vi "LDA CreateEmpty.vi"(8 "error in":errorcluster, 11 "numComponents":i32) -> (0 "error out":errorcluster, 3 "LDA":refnum<class "LDA.lvclass">)   [LabVIEW 2020, in "OpenLvVision_OpenCv.lvlib" / "LDA.lvclass"]
doc: "constructor Initializes a LDA with num_components (default 0)."
uses:
  LDA.lvclass
  C:/Users/lukas/Downloads/OpenLvVision_OpenCv/SourceCode/LabView/OpenLvVision_OpenCv/_LvHelpers/EdvrObject/EdvrObject.lvclass
  _LvHelpers/EdvrObject/TypeDef/Edvr.ctl
  _LvHelpers/EdvrObject/EdvrObject.lvclass/EdvrObject.ctl
  _LvHelpers/EdvrObject/EdvrObject.lvclass
  OpenLvVision_OpenCv.lvlib
  Dlls/OlvOpenCvWrapper.dll
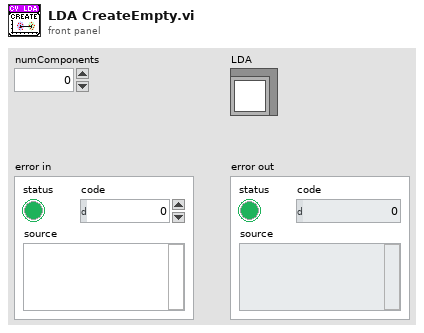
[diagram p1: front panel]
types:
  T1 = typedef "OpenLvVision_OpenCv.lvlib/EdvrObject.lvclass/Edvr.ctl" = refnum<data-value>
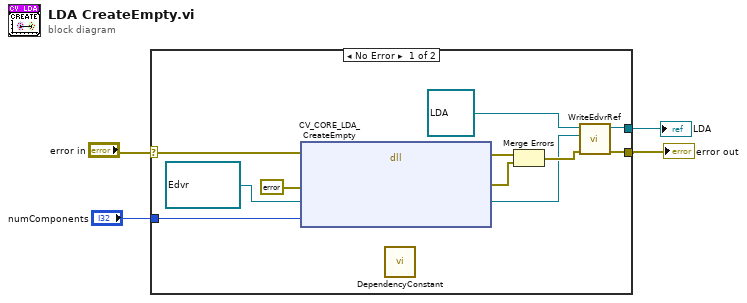
[diagram p0: block diagram]
diagram:
  n1 = case shown="No Error" "error in" {
    selector: "error in" -> [w12 w16]
    tunnel: [w14 w16] -> w3
    tunnel: [w15 _] -> w4
    tunnel: "numComponents" -> [w5 _]
    frame No Error {
      n2 = dll-call lib="C:/Users/lukas/Downloads/OpenLvVision_OpenCv/SourceCode/LabView/OpenLvVision_OpenCv/Dlls/OlvOpenCvWrapper.dll" fn="CV_CORE_LDA_CreateEmpty"(error in=w12, "Error"=errorcluster {"status"=FALSE, "code"=0, "source"=""} ("error out"), "edvrRef"=T1 refnum ("Edvr"), "numComponents"=w5) -> (error out=w10:errorcluster, "Error"=w6:errorcluster, "edvrRef"=w8:T1)  [unwired: 4 in, 1 out]
      n3 = call "DependencyConstant.vi"() -> ()  [unwired: 12 in]
      n4 = Merge Errors(w10, w6) -> (w9:errorcluster)
      n5 = call "WriteEdvrRef.vi"("error in (no error)"=w9, "Edvr"=w8, "EdvrObject in"=refnum<class "LDA.lvclass"> refnum ("OpenLvVision_OpenCv.lvlib:LDA")) -> ("error out"=w14:errorcluster, "EdvrObject out"=w15:refnum<class "LDA.lvclass">)  [unwired: 7 in]
    }
    frame Error {
    }
  }
  "error out" <- w3
  "LDA" <- w4
